vi "Qn5_Z.vi"(11 "String":string) -> (3 "Qn":dbl[](array[numeric]))   [LabVIEW 2015]
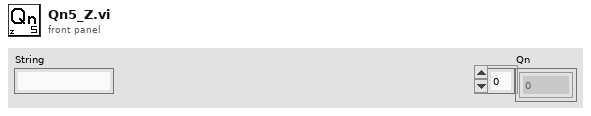
[diagram p1: front panel]
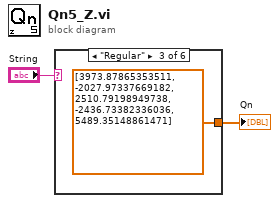
[diagram p0: block diagram]
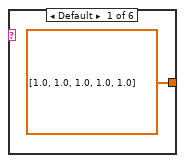
[diagram p2: hidden frame]
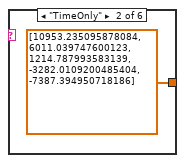
[diagram p3: hidden frame]
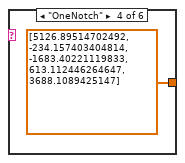
[diagram p4: hidden frame]
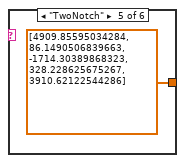
[diagram p5: hidden frame]
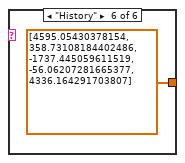
[diagram p6: hidden frame]
diagram:
  n1 = case shown="\"Regular\"" "String" {
    tunnel: [dbl[] [1.0, 1.0, 1.0, 1.0, 1.0] ("Qn") dbl[] [10953.235095878084, 6011.039747600123, 1214.787993583139, -3282.0109200485404, -7387.394950718186] ("Qn") dbl[] [3973.87865353511, -2027.97337669182, 2510.79198949738, -2436.73382336036, 5489.35148861471] ("Qn") dbl[] [5126.89514702492, -234.157403404814, -1683.40221119833, 613.112446264647, 3688.1089425147] ("Qn") dbl[] [4909.85595034284, 86.1490506839663, -1714.30389868323, 328.228625675267, 3910.62122544286] ("Qn") dbl[] [4595.05430378154, 358.73108184402486, -1737.445059611519, -56.06207281665377, 4336.164291703807] ("Qn")] -> w2
    frame Default {
    }
    frame "TimeOnly" {
    }
    frame "Regular" {
    }
    frame "OneNotch" {
    }
    frame "TwoNotch" {
    }
    frame "History" {
    }
  }
  "Qn" <- w2
